vi "main04.vi"() -> ()   [LabVIEW 2018]
uses:
  <vilib>/httpClient/LabVIEWHTTPClient.lvlib
panel:
  in  "탭 컨트롤":enum32{"관심 1", "관심 2", "관심 3", "관심 4", "관심 5"}(tab)
  in  "?":bool
  in  "품   번":string="034220"
  out "거래량":waveform(dbl)(graph)
  out "가격":waveform(i32)(graph)
  out "run":i32
  out "출력":T1
  in  "정지":bool
  in  "정지 2":bool
  out "출력 2":T1
  out "run 2":i32
  out "가격 2":waveform(i32)(graph)
  out "거래량 2":waveform(dbl)(graph)
  in  "품   번 2":string="005290"
  in  "?":bool
  in  "?":bool
  in  "?":bool
  in  "품   번 3":string="042700"
  out "거래량 3":waveform(dbl)(graph)
  out "가격 3":waveform(i32)(graph)
  out "run 3":i32
  out "출력 3":T1
  in  "정지 3":bool
  in  "품   번 4":string="046890"
  out "거래량 4":waveform(dbl)(graph)
  out "가격 4":waveform(i32)(graph)
  out "run 4":i32
  out "출력 4":T1
  in  "정지 4":bool
  in  "?":bool
  in  "?":bool
  in  "품   번 5":string="357780"
  out "거래량 5":waveform(dbl)(graph)
  out "가격 5":waveform(i32)(graph)
  out "run 5":i32
  out "출력 5":T1
  in  "정지 5":bool
  in  "품   번 6":string="012610"
  out "거래량 6":waveform(dbl)(graph)
  out "가격 6":waveform(i32)(graph)
  out "run 6":i32
  out "출력 6":T1
  in  "정지 6":bool
  in  "품   번 7":string="272450"
  out "거래량 7":waveform(dbl)(graph)
  out "가격 7":waveform(i32)(graph)
  out "run 7":i32
  out "출력 7":T1
  in  "정지 7":bool
  in  "품   번 8":string="003490"
  out "거래량 8":waveform(dbl)(graph)
  out "가격 8":waveform(i32)(graph)
  out "run 8":i32
  out "출력 8":T1
  in  "정지 8":bool
  in  "품   번 9":string="091580"
  out "거래량 9":waveform(dbl)(graph)
  out "가격 9":waveform(i32)(graph)
  out "run 9":i32
  out "출력 9":T1
  in  "정지 9":bool
  in  "품   번 10":string="089980"
  out "거래량 10":waveform(dbl)(graph)
  out "가격 10":waveform(i32)(graph)
  out "run 10":i32
  out "출력 10":T1
  in  "정지 10":bool
  in  "품   번 11":string="005070"
  out "거래량 11":waveform(dbl)(graph)
  out "가격 11":waveform(i32)(graph)
  out "run 11":i32
  out "출력 11":T1
  in  "정지 11":bool
  in  "품   번 12":string="078600"
  out "거래량 12":waveform(dbl)(graph)
  out "가격 12":waveform(i32)(graph)
  out "run 12":i32
  out "출력 12":T1
  in  "정지 12":bool
  in  "?":bool
  in  "?":bool
  in  "?":bool
  in  "?":bool
  in  "?":bool
  in  "?":bool
  in  "품   번 13":string="034220"
  out "거래량 13":waveform(dbl)(graph)
  out "가격 13":waveform(i32)(graph)
  out "run 13":i32
  out "출력 13":T1
  in  "정지 13":bool
  in  "품   번 14":string="039130"
  out "거래량 14":waveform(dbl)(graph)
  out "가격 14":waveform(i32)(graph)
  out "run 14":i32
  out "출력 14":T1
  in  "정지 14":bool
  in  "품   번 15":string="080160"
  out "거래량 15":waveform(dbl)(graph)
  out "가격 15":waveform(i32)(graph)
  out "run 15":i32
  out "출력 15":T1
  in  "정지 15":bool
  in  "품   번 16":string="020560"
  out "거래량 16":waveform(dbl)(graph)
  out "가격 16":waveform(i32)(graph)
  out "run 16":i32
  out "출력 16":T1
  in  "정지 16":bool
  in  "품   번 17":string="272450"
  out "거래량 17":waveform(dbl)(graph)
  out "가격 17":waveform(i32)(graph)
  out "run 17":i32
  out "출력 17":T1
  in  "정지 17":bool
  in  "품   번 18":string="003490"
  out "거래량 18":waveform(dbl)(graph)
  out "가격 18":waveform(i32)(graph)
  out "run 18":i32
  out "출력 18":T1
  in  "정지 18":bool
  in  "?":bool
  in  "?":bool
  in  "?":bool
  in  "?":bool
  in  "?":bool
  in  "?":bool
  in  "품   번 19":string="034220"
  out "거래량 19":waveform(dbl)(graph)
  out "가격 19":waveform(i32)(graph)
  out "run 19":i32
  out "출력 19":T1
  in  "정지 19":bool
  in  "품   번 20":string="034220"
  out "거래량 20":waveform(dbl)(graph)
  out "가격 20":waveform(i32)(graph)
  out "run 20":i32
  out "출력 20":T1
  in  "정지 20":bool
  in  "품   번 21":string="034220"
  out "거래량 21":waveform(dbl)(graph)
  out "가격 21":waveform(i32)(graph)
  out "run 21":i32
  out "출력 21":T1
  in  "정지 21":bool
  in  "품   번 22":string="034220"
  out "거래량 22":waveform(dbl)(graph)
  out "가격 22":waveform(i32)(graph)
  out "run 22":i32
  out "출력 22":T1
  in  "정지 22":bool
  in  "품   번 23":string="034220"
  out "거래량 23":waveform(dbl)(graph)
  out "가격 23":waveform(i32)(graph)
  out "run 23":i32
  out "출력 23":T1
  in  "정지 23":bool
  in  "품   번 24":string="034220"
  out "거래량 24":waveform(dbl)(graph)
  out "가격 24":waveform(i32)(graph)
  out "run 24":i32
  out "출력 24":T1
  in  "정지 24":bool
  in  "?":bool
  in  "?":bool
  in  "?":bool
  in  "?":bool
  in  "?":bool
  in  "?":bool
  in  "품   번 25":string="034220"
  out "거래량 25":waveform(dbl)(graph)
  out "가격 25":waveform(i32)(graph)
  out "run 25":i32
  out "출력 25":T1
  in  "정지 25":bool
  in  "품   번 26":string="034220"
  out "거래량 26":waveform(dbl)(graph)
  out "가격 26":waveform(i32)(graph)
  out "run 26":i32
  out "출력 26":T1
  in  "정지 26":bool
  in  "품   번 27":string="034220"
  out "거래량 27":waveform(dbl)(graph)
  out "가격 27":waveform(i32)(graph)
  out "run 27":i32
  out "출력 27":T1
  in  "정지 27":bool
  in  "품   번 28":string="034220"
  out "거래량 28":waveform(dbl)(graph)
  out "가격 28":waveform(i32)(graph)
  out "run 28":i32
  out "출력 28":T1
  in  "정지 28":bool
  in  "품   번 29":string="034220"
  out "거래량 29":waveform(dbl)(graph)
  out "가격 29":waveform(i32)(graph)
  out "run 29":i32
  out "출력 29":T1
  in  "정지 29":bool
  in  "품   번 30":string="034220"
  out "거래량 30":waveform(dbl)(graph)
  out "가격 30":waveform(i32)(graph)
  out "run 30":i32
  out "출력 30":T1
  in  "정지 30":bool
  in  "?":bool
  in  "?":bool
  in  "?":bool
  in  "?":bool
  in  "?":bool
  in  "?":bool
  # "Naver 주식 데이터 가져오기"
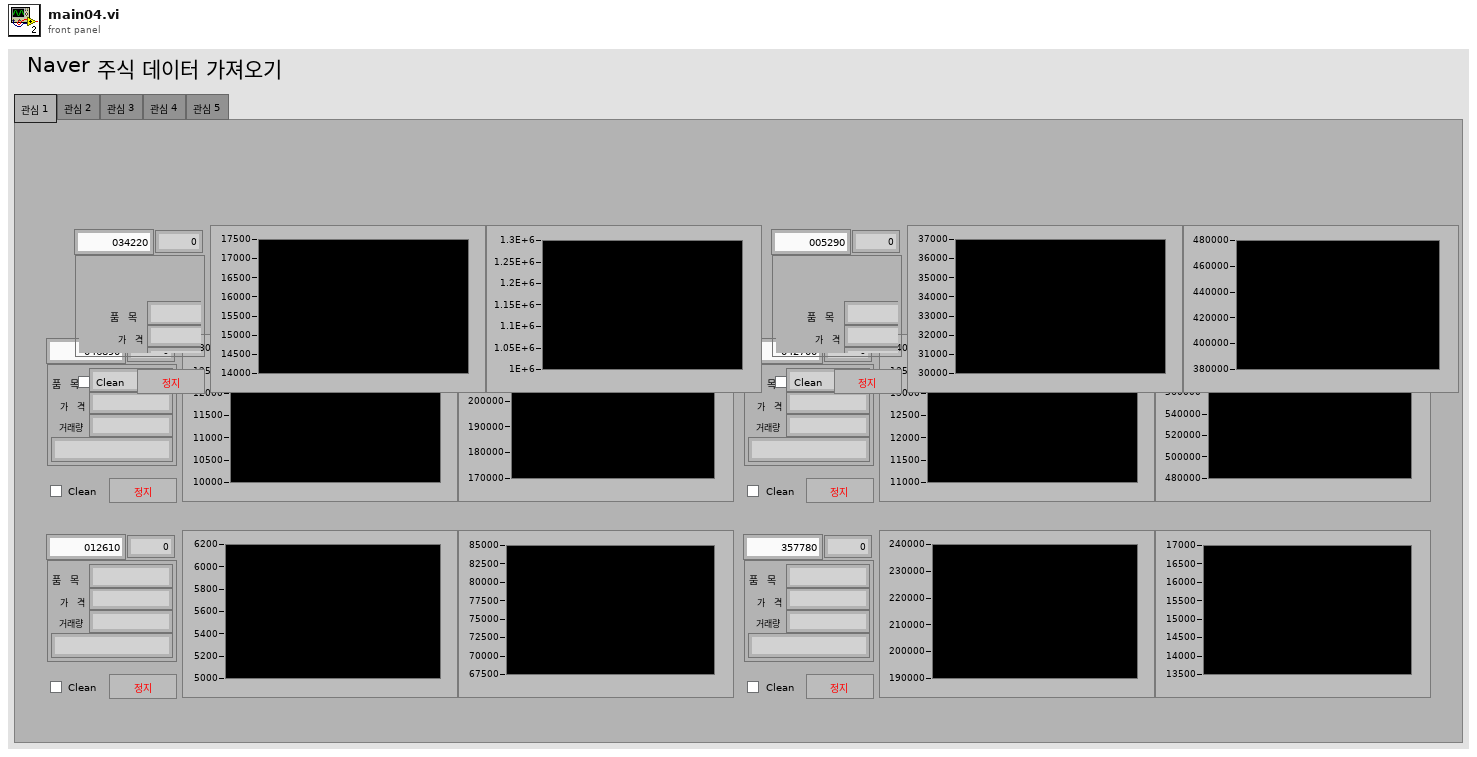
[diagram p1: front panel]
types:
  T1 = cluster{"품   목":string, "가   격":i32, "거래량":dbl, "일시":string}
  T2 = typedef "LabVIEWHTTPClient.lvlib/ClientHandle.ctl" = refnum<k1>
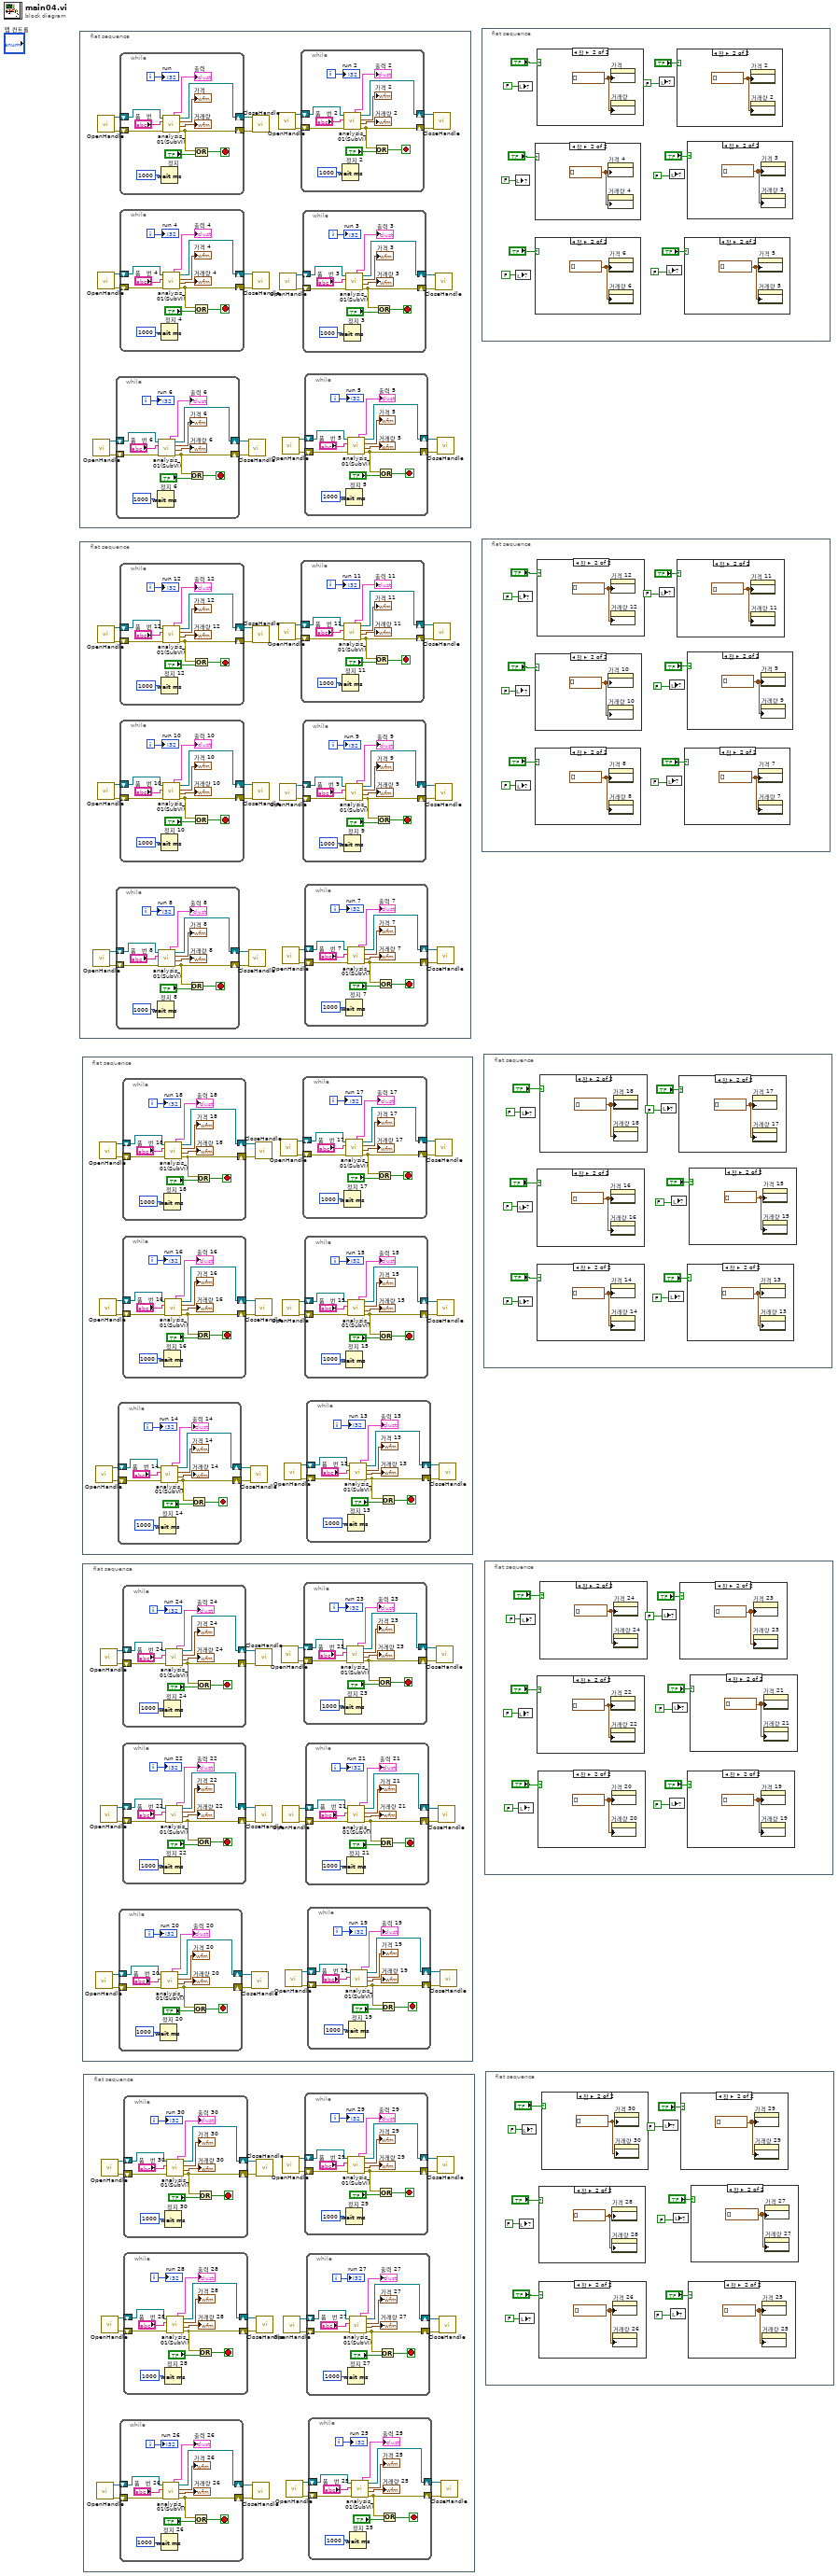
[diagram p0: block diagram]
diagram:
  n1 = flat-sequence {
    frame #0 {
      n2 = call <vilib>:"OpenHandle.vi"() -> ("client handle out"=w5:T2, "error out"=w6:errorcluster)  [unwired: 14 in]
      n3 = call <vilib>:"OpenHandle.vi"() -> ("client handle out"=w21:T2, "error out"=w22:errorcluster)  [unwired: 14 in]
      n4 = call <vilib>:"OpenHandle.vi"() -> ("client handle out"=w12:T2, "error out"=w11:errorcluster)  [unwired: 14 in]
      n5 = while {
        shift-right: [w46] -> w7
        shift-left: w5 -> [w47]
        shift-right: [w44] -> w8
        shift-left: w6 -> [w45]
        i -> [w41]
        stop <- w42 stop-if-true
        n6 = Wait (ms)(milliseconds to wait=u32 1000 ("대기 시간 (ms)")) -> ()  [unwired: 1 out]
        n7 = call "analysis_01(SubVI).vi"("에러 입력(에러 없음)"=w45, "품   번"="품   번 6", "참조 번호 입력"=w47) -> ("에러 출력"=w44:errorcluster, "거래량"=→"거래량 6":waveform(dbl), "가격"=→"가격 6":waveform(i32), "참조 번호 출력"=w46:T2, "출력"=→"출력 6":T1)  [unwired: 4 in]
        n8 = Or(x=w44, y="정지 6") -> (x .or. y?=w42:bool)
        "run 6" <- w41
      }
      n9 = while {
        shift-right: [w94] -> w23
        shift-left: w21 -> [w95]
        shift-right: [w92] -> w24
        shift-left: w22 -> [w93]
        i -> [w89]
        stop <- w90 stop-if-true
        n10 = Wait (ms)(milliseconds to wait=u32 1000 ("대기 시간 (ms)")) -> ()  [unwired: 1 out]
        n11 = call "analysis_01(SubVI).vi"("에러 입력(에러 없음)"=w93, "품   번"="품   번", "참조 번호 입력"=w95) -> ("에러 출력"=w92:errorcluster, "거래량"=→"거래량":waveform(dbl), "가격"=→"가격":waveform(i32), "참조 번호 출력"=w94:T2, "출력"=→"출력":T1)  [unwired: 4 in]
        n12 = Or(x=w92, y="정지") -> (x .or. y?=w90:bool)
        "run" <- w89
      }
      n13 = while {
        shift-right: [w70] -> w10
        shift-left: w12 -> [w71]
        shift-right: [w68] -> w9
        shift-left: w11 -> [w69]
        i -> [w65]
        stop <- w66 stop-if-true
        n14 = Wait (ms)(milliseconds to wait=u32 1000 ("대기 시간 (ms)")) -> ()  [unwired: 1 out]
        n15 = call "analysis_01(SubVI).vi"("에러 입력(에러 없음)"=w69, "품   번"="품   번 4", "참조 번호 입력"=w71) -> ("에러 출력"=w68:errorcluster, "거래량"=→"거래량 4":waveform(dbl), "가격"=→"가격 4":waveform(i32), "참조 번호 출력"=w70:T2, "출력"=→"출력 4":T1)  [unwired: 4 in]
        n16 = Or(x=w68, y="정지 4") -> (x .or. y?=w66:bool)
        "run 4" <- w65
      }
      n17 = call <vilib>:"CloseHandle.vi"("client handle"=w7, "error in (no error)"=w8) -> ()  [unwired: 13 in, 1 out]
      n18 = call <vilib>:"CloseHandle.vi"("client handle"=w23, "error in (no error)"=w24) -> ()  [unwired: 13 in, 1 out]
      n19 = call <vilib>:"CloseHandle.vi"("client handle"=w10, "error in (no error)"=w9) -> ()  [unwired: 13 in, 1 out]
      n20 = call <vilib>:"OpenHandle.vi"() -> ("client handle out"=w20:T2, "error out"=w19:errorcluster)  [unwired: 14 in]
      n21 = call <vilib>:"OpenHandle.vi"() -> ("client handle out"=w13:T2, "error out"=w14:errorcluster)  [unwired: 14 in]
      n22 = call <vilib>:"OpenHandle.vi"() -> ("client handle out"=w4:T2, "error out"=w3:errorcluster)  [unwired: 14 in]
      n23 = while {
        shift-right: [w82] -> w18
        shift-left: w20 -> [w83]
        shift-right: [w80] -> w17
        shift-left: w19 -> [w81]
        i -> [w77]
        stop <- w78 stop-if-true
        n24 = Wait (ms)(milliseconds to wait=u32 1000 ("대기 시간 (ms)")) -> ()  [unwired: 1 out]
        n25 = call "analysis_01(SubVI).vi"("에러 입력(에러 없음)"=w81, "품   번"="품   번 2", "참조 번호 입력"=w83) -> ("에러 출력"=w80:errorcluster, "거래량"=→"거래량 2":waveform(dbl), "가격"=→"가격 2":waveform(i32), "참조 번호 출력"=w82:T2, "출력"=→"출력 2":T1)  [unwired: 4 in]
        n26 = Or(x=w80, y="정지 2") -> (x .or. y?=w78:bool)
        "run 2" <- w77
      }
      n27 = while {
        shift-right: [w58] -> w15
        shift-left: w13 -> [w59]
        shift-right: [w56] -> w16
        shift-left: w14 -> [w57]
        i -> [w53]
        stop <- w54 stop-if-true
        n28 = Wait (ms)(milliseconds to wait=u32 1000 ("대기 시간 (ms)")) -> ()  [unwired: 1 out]
        n29 = call "analysis_01(SubVI).vi"("에러 입력(에러 없음)"=w57, "품   번"="품   번 3", "참조 번호 입력"=w59) -> ("에러 출력"=w56:errorcluster, "거래량"=→"거래량 3":waveform(dbl), "가격"=→"가격 3":waveform(i32), "참조 번호 출력"=w58:T2, "출력"=→"출력 3":T1)  [unwired: 4 in]
        n30 = Or(x=w56, y="정지 3") -> (x .or. y?=w54:bool)
        "run 3" <- w53
      }
      n31 = while {
        shift-right: [w34] -> w2
        shift-left: w4 -> [w35]
        shift-right: [w32] -> w1
        shift-left: w3 -> [w33]
        i -> [w29]
        stop <- w30 stop-if-true
        n32 = Wait (ms)(milliseconds to wait=u32 1000 ("대기 시간 (ms)")) -> ()  [unwired: 1 out]
        n33 = call "analysis_01(SubVI).vi"("에러 입력(에러 없음)"=w33, "품   번"="품   번 5", "참조 번호 입력"=w35) -> ("에러 출력"=w32:errorcluster, "거래량"=→"거래량 5":waveform(dbl), "가격"=→"가격 5":waveform(i32), "참조 번호 출력"=w34:T2, "출력"=→"출력 5":T1)  [unwired: 4 in]
        n34 = Or(x=w32, y="정지 5") -> (x .or. y?=w30:bool)
        "run 5" <- w29
      }
      n35 = call <vilib>:"CloseHandle.vi"("client handle"=w18, "error in (no error)"=w17) -> ()  [unwired: 13 in, 1 out]
      n36 = call <vilib>:"CloseHandle.vi"("client handle"=w15, "error in (no error)"=w16) -> ()  [unwired: 13 in, 1 out]
      n37 = call <vilib>:"CloseHandle.vi"("client handle"=w2, "error in (no error)"=w1) -> ()  [unwired: 13 in, 1 out]
    }
  }
  n38 = flat-sequence {
    frame #0 {
      n39 = call <vilib>:"OpenHandle.vi"() -> ("client handle out"=w101:T2, "error out"=w102:errorcluster)  [unwired: 14 in]
      n40 = call <vilib>:"OpenHandle.vi"() -> ("client handle out"=w117:T2, "error out"=w118:errorcluster)  [unwired: 14 in]
      n41 = call <vilib>:"OpenHandle.vi"() -> ("client handle out"=w108:T2, "error out"=w107:errorcluster)  [unwired: 14 in]
      n42 = while {
        shift-right: [w142] -> w103
        shift-left: w101 -> [w143]
        shift-right: [w140] -> w104
        shift-left: w102 -> [w141]
        i -> [w137]
        stop <- w138 stop-if-true
        n43 = Wait (ms)(milliseconds to wait=u32 1000 ("대기 시간 (ms)")) -> ()  [unwired: 1 out]
        n44 = call "analysis_01(SubVI).vi"("에러 입력(에러 없음)"=w141, "품   번"="품   번 8", "참조 번호 입력"=w143) -> ("에러 출력"=w140:errorcluster, "거래량"=→"거래량 8":waveform(dbl), "가격"=→"가격 8":waveform(i32), "참조 번호 출력"=w142:T2, "출력"=→"출력 8":T1)  [unwired: 4 in]
        n45 = Or(x=w140, y="정지 8") -> (x .or. y?=w138:bool)
        "run 8" <- w137
      }
      n46 = while {
        shift-right: [w190] -> w119
        shift-left: w117 -> [w191]
        shift-right: [w188] -> w120
        shift-left: w118 -> [w189]
        i -> [w185]
        stop <- w186 stop-if-true
        n47 = Wait (ms)(milliseconds to wait=u32 1000 ("대기 시간 (ms)")) -> ()  [unwired: 1 out]
        n48 = call "analysis_01(SubVI).vi"("에러 입력(에러 없음)"=w189, "품   번"="품   번 12", "참조 번호 입력"=w191) -> ("에러 출력"=w188:errorcluster, "거래량"=→"거래량 12":waveform(dbl), "가격"=→"가격 12":waveform(i32), "참조 번호 출력"=w190:T2, "출력"=→"출력 12":T1)  [unwired: 4 in]
        n49 = Or(x=w188, y="정지 12") -> (x .or. y?=w186:bool)
        "run 12" <- w185
      }
      n50 = while {
        shift-right: [w166] -> w106
        shift-left: w108 -> [w167]
        shift-right: [w164] -> w105
        shift-left: w107 -> [w165]
        i -> [w161]
        stop <- w162 stop-if-true
        n51 = Wait (ms)(milliseconds to wait=u32 1000 ("대기 시간 (ms)")) -> ()  [unwired: 1 out]
        n52 = call "analysis_01(SubVI).vi"("에러 입력(에러 없음)"=w165, "품   번"="품   번 10", "참조 번호 입력"=w167) -> ("에러 출력"=w164:errorcluster, "거래량"=→"거래량 10":waveform(dbl), "가격"=→"가격 10":waveform(i32), "참조 번호 출력"=w166:T2, "출력"=→"출력 10":T1)  [unwired: 4 in]
        n53 = Or(x=w164, y="정지 10") -> (x .or. y?=w162:bool)
        "run 10" <- w161
      }
      n54 = call <vilib>:"CloseHandle.vi"("client handle"=w103, "error in (no error)"=w104) -> ()  [unwired: 13 in, 1 out]
      n55 = call <vilib>:"CloseHandle.vi"("client handle"=w119, "error in (no error)"=w120) -> ()  [unwired: 13 in, 1 out]
      n56 = call <vilib>:"CloseHandle.vi"("client handle"=w106, "error in (no error)"=w105) -> ()  [unwired: 13 in, 1 out]
      n57 = call <vilib>:"OpenHandle.vi"() -> ("client handle out"=w116:T2, "error out"=w115:errorcluster)  [unwired: 14 in]
      n58 = call <vilib>:"OpenHandle.vi"() -> ("client handle out"=w109:T2, "error out"=w110:errorcluster)  [unwired: 14 in]
      n59 = call <vilib>:"OpenHandle.vi"() -> ("client handle out"=w100:T2, "error out"=w99:errorcluster)  [unwired: 14 in]
      n60 = while {
        shift-right: [w178] -> w114
        shift-left: w116 -> [w179]
        shift-right: [w176] -> w113
        shift-left: w115 -> [w177]
        i -> [w173]
        stop <- w174 stop-if-true
        n61 = Wait (ms)(milliseconds to wait=u32 1000 ("대기 시간 (ms)")) -> ()  [unwired: 1 out]
        n62 = call "analysis_01(SubVI).vi"("에러 입력(에러 없음)"=w177, "품   번"="품   번 11", "참조 번호 입력"=w179) -> ("에러 출력"=w176:errorcluster, "거래량"=→"거래량 11":waveform(dbl), "가격"=→"가격 11":waveform(i32), "참조 번호 출력"=w178:T2, "출력"=→"출력 11":T1)  [unwired: 4 in]
        n63 = Or(x=w176, y="정지 11") -> (x .or. y?=w174:bool)
        "run 11" <- w173
      }
      n64 = while {
        shift-right: [w154] -> w111
        shift-left: w109 -> [w155]
        shift-right: [w152] -> w112
        shift-left: w110 -> [w153]
        i -> [w149]
        stop <- w150 stop-if-true
        n65 = Wait (ms)(milliseconds to wait=u32 1000 ("대기 시간 (ms)")) -> ()  [unwired: 1 out]
        n66 = call "analysis_01(SubVI).vi"("에러 입력(에러 없음)"=w153, "품   번"="품   번 9", "참조 번호 입력"=w155) -> ("에러 출력"=w152:errorcluster, "거래량"=→"거래량 9":waveform(dbl), "가격"=→"가격 9":waveform(i32), "참조 번호 출력"=w154:T2, "출력"=→"출력 9":T1)  [unwired: 4 in]
        n67 = Or(x=w152, y="정지 9") -> (x .or. y?=w150:bool)
        "run 9" <- w149
      }
      n68 = while {
        shift-right: [w130] -> w98
        shift-left: w100 -> [w131]
        shift-right: [w128] -> w97
        shift-left: w99 -> [w129]
        i -> [w125]
        stop <- w126 stop-if-true
        n69 = Wait (ms)(milliseconds to wait=u32 1000 ("대기 시간 (ms)")) -> ()  [unwired: 1 out]
        n70 = call "analysis_01(SubVI).vi"("에러 입력(에러 없음)"=w129, "품   번"="품   번 7", "참조 번호 입력"=w131) -> ("에러 출력"=w128:errorcluster, "거래량"=→"거래량 7":waveform(dbl), "가격"=→"가격 7":waveform(i32), "참조 번호 출력"=w130:T2, "출력"=→"출력 7":T1)  [unwired: 4 in]
        n71 = Or(x=w128, y="정지 7") -> (x .or. y?=w126:bool)
        "run 7" <- w125
      }
      n72 = call <vilib>:"CloseHandle.vi"("client handle"=w114, "error in (no error)"=w113) -> ()  [unwired: 13 in, 1 out]
      n73 = call <vilib>:"CloseHandle.vi"("client handle"=w111, "error in (no error)"=w112) -> ()  [unwired: 13 in, 1 out]
      n74 = call <vilib>:"CloseHandle.vi"("client handle"=w98, "error in (no error)"=w97) -> ()  [unwired: 13 in, 1 out]
    }
  }
  n75 = flat-sequence {
    frame #0 {
      n76 = call <vilib>:"OpenHandle.vi"() -> ("client handle out"=w197:T2, "error out"=w198:errorcluster)  [unwired: 14 in]
      n77 = call <vilib>:"OpenHandle.vi"() -> ("client handle out"=w213:T2, "error out"=w214:errorcluster)  [unwired: 14 in]
      n78 = call <vilib>:"OpenHandle.vi"() -> ("client handle out"=w204:T2, "error out"=w203:errorcluster)  [unwired: 14 in]
      n79 = while {
        shift-right: [w238] -> w199
        shift-left: w197 -> [w239]
        shift-right: [w236] -> w200
        shift-left: w198 -> [w237]
        i -> [w233]
        stop <- w234 stop-if-true
        n80 = Wait (ms)(milliseconds to wait=u32 1000 ("대기 시간 (ms)")) -> ()  [unwired: 1 out]
        n81 = call "analysis_01(SubVI).vi"("에러 입력(에러 없음)"=w237, "품   번"="품   번 14", "참조 번호 입력"=w239) -> ("에러 출력"=w236:errorcluster, "거래량"=→"거래량 14":waveform(dbl), "가격"=→"가격 14":waveform(i32), "참조 번호 출력"=w238:T2, "출력"=→"출력 14":T1)  [unwired: 4 in]
        n82 = Or(x=w236, y="정지 14") -> (x .or. y?=w234:bool)
        "run 14" <- w233
      }
      n83 = while {
        shift-right: [w286] -> w215
        shift-left: w213 -> [w287]
        shift-right: [w284] -> w216
        shift-left: w214 -> [w285]
        i -> [w281]
        stop <- w282 stop-if-true
        n84 = Wait (ms)(milliseconds to wait=u32 1000 ("대기 시간 (ms)")) -> ()  [unwired: 1 out]
        n85 = call "analysis_01(SubVI).vi"("에러 입력(에러 없음)"=w285, "품   번"="품   번 18", "참조 번호 입력"=w287) -> ("에러 출력"=w284:errorcluster, "거래량"=→"거래량 18":waveform(dbl), "가격"=→"가격 18":waveform(i32), "참조 번호 출력"=w286:T2, "출력"=→"출력 18":T1)  [unwired: 4 in]
        n86 = Or(x=w284, y="정지 18") -> (x .or. y?=w282:bool)
        "run 18" <- w281
      }
      n87 = while {
        shift-right: [w262] -> w202
        shift-left: w204 -> [w263]
        shift-right: [w260] -> w201
        shift-left: w203 -> [w261]
        i -> [w257]
        stop <- w258 stop-if-true
        n88 = Wait (ms)(milliseconds to wait=u32 1000 ("대기 시간 (ms)")) -> ()  [unwired: 1 out]
        n89 = call "analysis_01(SubVI).vi"("에러 입력(에러 없음)"=w261, "품   번"="품   번 16", "참조 번호 입력"=w263) -> ("에러 출력"=w260:errorcluster, "거래량"=→"거래량 16":waveform(dbl), "가격"=→"가격 16":waveform(i32), "참조 번호 출력"=w262:T2, "출력"=→"출력 16":T1)  [unwired: 4 in]
        n90 = Or(x=w260, y="정지 16") -> (x .or. y?=w258:bool)
        "run 16" <- w257
      }
      n91 = call <vilib>:"CloseHandle.vi"("client handle"=w199, "error in (no error)"=w200) -> ()  [unwired: 13 in, 1 out]
      n92 = call <vilib>:"CloseHandle.vi"("client handle"=w215, "error in (no error)"=w216) -> ()  [unwired: 13 in, 1 out]
      n93 = call <vilib>:"CloseHandle.vi"("client handle"=w202, "error in (no error)"=w201) -> ()  [unwired: 13 in, 1 out]
      n94 = call <vilib>:"OpenHandle.vi"() -> ("client handle out"=w212:T2, "error out"=w211:errorcluster)  [unwired: 14 in]
      n95 = call <vilib>:"OpenHandle.vi"() -> ("client handle out"=w205:T2, "error out"=w206:errorcluster)  [unwired: 14 in]
      n96 = call <vilib>:"OpenHandle.vi"() -> ("client handle out"=w196:T2, "error out"=w195:errorcluster)  [unwired: 14 in]
      n97 = while {
        shift-right: [w274] -> w210
        shift-left: w212 -> [w275]
        shift-right: [w272] -> w209
        shift-left: w211 -> [w273]
        i -> [w269]
        stop <- w270 stop-if-true
        n98 = Wait (ms)(milliseconds to wait=u32 1000 ("대기 시간 (ms)")) -> ()  [unwired: 1 out]
        n99 = call "analysis_01(SubVI).vi"("에러 입력(에러 없음)"=w273, "품   번"="품   번 17", "참조 번호 입력"=w275) -> ("에러 출력"=w272:errorcluster, "거래량"=→"거래량 17":waveform(dbl), "가격"=→"가격 17":waveform(i32), "참조 번호 출력"=w274:T2, "출력"=→"출력 17":T1)  [unwired: 4 in]
        n100 = Or(x=w272, y="정지 17") -> (x .or. y?=w270:bool)
        "run 17" <- w269
      }
      n101 = while {
        shift-right: [w250] -> w207
        shift-left: w205 -> [w251]
        shift-right: [w248] -> w208
        shift-left: w206 -> [w249]
        i -> [w245]
        stop <- w246 stop-if-true
        n102 = Wait (ms)(milliseconds to wait=u32 1000 ("대기 시간 (ms)")) -> ()  [unwired: 1 out]
        n103 = call "analysis_01(SubVI).vi"("에러 입력(에러 없음)"=w249, "품   번"="품   번 15", "참조 번호 입력"=w251) -> ("에러 출력"=w248:errorcluster, "거래량"=→"거래량 15":waveform(dbl), "가격"=→"가격 15":waveform(i32), "참조 번호 출력"=w250:T2, "출력"=→"출력 15":T1)  [unwired: 4 in]
        n104 = Or(x=w248, y="정지 15") -> (x .or. y?=w246:bool)
        "run 15" <- w245
      }
      n105 = while {
        shift-right: [w226] -> w194
        shift-left: w196 -> [w227]
        shift-right: [w224] -> w193
        shift-left: w195 -> [w225]
        i -> [w221]
        stop <- w222 stop-if-true
        n106 = Wait (ms)(milliseconds to wait=u32 1000 ("대기 시간 (ms)")) -> ()  [unwired: 1 out]
        n107 = call "analysis_01(SubVI).vi"("에러 입력(에러 없음)"=w225, "품   번"="품   번 13", "참조 번호 입력"=w227) -> ("에러 출력"=w224:errorcluster, "거래량"=→"거래량 13":waveform(dbl), "가격"=→"가격 13":waveform(i32), "참조 번호 출력"=w226:T2, "출력"=→"출력 13":T1)  [unwired: 4 in]
        n108 = Or(x=w224, y="정지 13") -> (x .or. y?=w222:bool)
        "run 13" <- w221
      }
      n109 = call <vilib>:"CloseHandle.vi"("client handle"=w210, "error in (no error)"=w209) -> ()  [unwired: 13 in, 1 out]
      n110 = call <vilib>:"CloseHandle.vi"("client handle"=w207, "error in (no error)"=w208) -> ()  [unwired: 13 in, 1 out]
      n111 = call <vilib>:"CloseHandle.vi"("client handle"=w194, "error in (no error)"=w193) -> ()  [unwired: 13 in, 1 out]
    }
  }
  n112 = flat-sequence {
    frame #0 {
      n113 = call <vilib>:"OpenHandle.vi"() -> ("client handle out"=w293:T2, "error out"=w294:errorcluster)  [unwired: 14 in]
      n114 = call <vilib>:"OpenHandle.vi"() -> ("client handle out"=w309:T2, "error out"=w310:errorcluster)  [unwired: 14 in]
      n115 = call <vilib>:"OpenHandle.vi"() -> ("client handle out"=w300:T2, "error out"=w299:errorcluster)  [unwired: 14 in]
      n116 = while {
        shift-right: [w334] -> w295
        shift-left: w293 -> [w335]
        shift-right: [w332] -> w296
        shift-left: w294 -> [w333]
        i -> [w329]
        stop <- w330 stop-if-true
        n117 = Wait (ms)(milliseconds to wait=u32 1000 ("대기 시간 (ms)")) -> ()  [unwired: 1 out]
        n118 = call "analysis_01(SubVI).vi"("에러 입력(에러 없음)"=w333, "품   번"="품   번 20", "참조 번호 입력"=w335) -> ("에러 출력"=w332:errorcluster, "거래량"=→"거래량 20":waveform(dbl), "가격"=→"가격 20":waveform(i32), "참조 번호 출력"=w334:T2, "출력"=→"출력 20":T1)  [unwired: 4 in]
        n119 = Or(x=w332, y="정지 20") -> (x .or. y?=w330:bool)
        "run 20" <- w329
      }
      n120 = while {
        shift-right: [w382] -> w311
        shift-left: w309 -> [w383]
        shift-right: [w380] -> w312
        shift-left: w310 -> [w381]
        i -> [w377]
        stop <- w378 stop-if-true
        n121 = Wait (ms)(milliseconds to wait=u32 1000 ("대기 시간 (ms)")) -> ()  [unwired: 1 out]
        n122 = call "analysis_01(SubVI).vi"("에러 입력(에러 없음)"=w381, "품   번"="품   번 24", "참조 번호 입력"=w383) -> ("에러 출력"=w380:errorcluster, "거래량"=→"거래량 24":waveform(dbl), "가격"=→"가격 24":waveform(i32), "참조 번호 출력"=w382:T2, "출력"=→"출력 24":T1)  [unwired: 4 in]
        n123 = Or(x=w380, y="정지 24") -> (x .or. y?=w378:bool)
        "run 24" <- w377
      }
      n124 = while {
        shift-right: [w358] -> w298
        shift-left: w300 -> [w359]
        shift-right: [w356] -> w297
        shift-left: w299 -> [w357]
        i -> [w353]
        stop <- w354 stop-if-true
        n125 = Wait (ms)(milliseconds to wait=u32 1000 ("대기 시간 (ms)")) -> ()  [unwired: 1 out]
        n126 = call "analysis_01(SubVI).vi"("에러 입력(에러 없음)"=w357, "품   번"="품   번 22", "참조 번호 입력"=w359) -> ("에러 출력"=w356:errorcluster, "거래량"=→"거래량 22":waveform(dbl), "가격"=→"가격 22":waveform(i32), "참조 번호 출력"=w358:T2, "출력"=→"출력 22":T1)  [unwired: 4 in]
        n127 = Or(x=w356, y="정지 22") -> (x .or. y?=w354:bool)
        "run 22" <- w353
      }
      n128 = call <vilib>:"CloseHandle.vi"("client handle"=w295, "error in (no error)"=w296) -> ()  [unwired: 13 in, 1 out]
      n129 = call <vilib>:"CloseHandle.vi"("client handle"=w311, "error in (no error)"=w312) -> ()  [unwired: 13 in, 1 out]
      n130 = call <vilib>:"CloseHandle.vi"("client handle"=w298, "error in (no error)"=w297) -> ()  [unwired: 13 in, 1 out]
      n131 = call <vilib>:"OpenHandle.vi"() -> ("client handle out"=w308:T2, "error out"=w307:errorcluster)  [unwired: 14 in]
      n132 = call <vilib>:"OpenHandle.vi"() -> ("client handle out"=w301:T2, "error out"=w302:errorcluster)  [unwired: 14 in]
      n133 = call <vilib>:"OpenHandle.vi"() -> ("client handle out"=w292:T2, "error out"=w291:errorcluster)  [unwired: 14 in]
      n134 = while {
        shift-right: [w370] -> w306
        shift-left: w308 -> [w371]
        shift-right: [w368] -> w305
        shift-left: w307 -> [w369]
        i -> [w365]
        stop <- w366 stop-if-true
        n135 = Wait (ms)(milliseconds to wait=u32 1000 ("대기 시간 (ms)")) -> ()  [unwired: 1 out]
        n136 = call "analysis_01(SubVI).vi"("에러 입력(에러 없음)"=w369, "품   번"="품   번 23", "참조 번호 입력"=w371) -> ("에러 출력"=w368:errorcluster, "거래량"=→"거래량 23":waveform(dbl), "가격"=→"가격 23":waveform(i32), "참조 번호 출력"=w370:T2, "출력"=→"출력 23":T1)  [unwired: 4 in]
        n137 = Or(x=w368, y="정지 23") -> (x .or. y?=w366:bool)
        "run 23" <- w365
      }
      n138 = while {
        shift-right: [w346] -> w303
        shift-left: w301 -> [w347]
        shift-right: [w344] -> w304
        shift-left: w302 -> [w345]
        i -> [w341]
        stop <- w342 stop-if-true
        n139 = Wait (ms)(milliseconds to wait=u32 1000 ("대기 시간 (ms)")) -> ()  [unwired: 1 out]
        n140 = call "analysis_01(SubVI).vi"("에러 입력(에러 없음)"=w345, "품   번"="품   번 21", "참조 번호 입력"=w347) -> ("에러 출력"=w344:errorcluster, "거래량"=→"거래량 21":waveform(dbl), "가격"=→"가격 21":waveform(i32), "참조 번호 출력"=w346:T2, "출력"=→"출력 21":T1)  [unwired: 4 in]
        n141 = Or(x=w344, y="정지 21") -> (x .or. y?=w342:bool)
        "run 21" <- w341
      }
      n142 = while {
        shift-right: [w322] -> w290
        shift-left: w292 -> [w323]
        shift-right: [w320] -> w289
        shift-left: w291 -> [w321]
        i -> [w317]
        stop <- w318 stop-if-true
        n143 = Wait (ms)(milliseconds to wait=u32 1000 ("대기 시간 (ms)")) -> ()  [unwired: 1 out]
        n144 = call "analysis_01(SubVI).vi"("에러 입력(에러 없음)"=w321, "품   번"="품   번 19", "참조 번호 입력"=w323) -> ("에러 출력"=w320:errorcluster, "거래량"=→"거래량 19":waveform(dbl), "가격"=→"가격 19":waveform(i32), "참조 번호 출력"=w322:T2, "출력"=→"출력 19":T1)  [unwired: 4 in]
        n145 = Or(x=w320, y="정지 19") -> (x .or. y?=w318:bool)
        "run 19" <- w317
      }
      n146 = call <vilib>:"CloseHandle.vi"("client handle"=w306, "error in (no error)"=w305) -> ()  [unwired: 13 in, 1 out]
      n147 = call <vilib>:"CloseHandle.vi"("client handle"=w303, "error in (no error)"=w304) -> ()  [unwired: 13 in, 1 out]
      n148 = call <vilib>:"CloseHandle.vi"("client handle"=w290, "error in (no error)"=w289) -> ()  [unwired: 13 in, 1 out]
    }
  }
  n149 = flat-sequence {
    frame #0 {
      n150 = call <vilib>:"OpenHandle.vi"() -> ("client handle out"=w389:T2, "error out"=w390:errorcluster)  [unwired: 14 in]
      n151 = call <vilib>:"OpenHandle.vi"() -> ("client handle out"=w405:T2, "error out"=w406:errorcluster)  [unwired: 14 in]
      n152 = call <vilib>:"OpenHandle.vi"() -> ("client handle out"=w396:T2, "error out"=w395:errorcluster)  [unwired: 14 in]
      n153 = while {
        shift-right: [w430] -> w391
        shift-left: w389 -> [w431]
        shift-right: [w428] -> w392
        shift-left: w390 -> [w429]
        i -> [w425]
        stop <- w426 stop-if-true
        n154 = Wait (ms)(milliseconds to wait=u32 1000 ("대기 시간 (ms)")) -> ()  [unwired: 1 out]
        n155 = call "analysis_01(SubVI).vi"("에러 입력(에러 없음)"=w429, "품   번"="품   번 26", "참조 번호 입력"=w431) -> ("에러 출력"=w428:errorcluster, "거래량"=→"거래량 26":waveform(dbl), "가격"=→"가격 26":waveform(i32), "참조 번호 출력"=w430:T2, "출력"=→"출력 26":T1)  [unwired: 4 in]
        n156 = Or(x=w428, y="정지 26") -> (x .or. y?=w426:bool)
        "run 26" <- w425
      }
      n157 = while {
        shift-right: [w478] -> w407
        shift-left: w405 -> [w479]
        shift-right: [w476] -> w408
        shift-left: w406 -> [w477]
        i -> [w473]
        stop <- w474 stop-if-true
        n158 = Wait (ms)(milliseconds to wait=u32 1000 ("대기 시간 (ms)")) -> ()  [unwired: 1 out]
        n159 = call "analysis_01(SubVI).vi"("에러 입력(에러 없음)"=w477, "품   번"="품   번 30", "참조 번호 입력"=w479) -> ("에러 출력"=w476:errorcluster, "거래량"=→"거래량 30":waveform(dbl), "가격"=→"가격 30":waveform(i32), "참조 번호 출력"=w478:T2, "출력"=→"출력 30":T1)  [unwired: 4 in]
        n160 = Or(x=w476, y="정지 30") -> (x .or. y?=w474:bool)
        "run 30" <- w473
      }
      n161 = while {
        shift-right: [w454] -> w394
        shift-left: w396 -> [w455]
        shift-right: [w452] -> w393
        shift-left: w395 -> [w453]
        i -> [w449]
        stop <- w450 stop-if-true
        n162 = Wait (ms)(milliseconds to wait=u32 1000 ("대기 시간 (ms)")) -> ()  [unwired: 1 out]
        n163 = call "analysis_01(SubVI).vi"("에러 입력(에러 없음)"=w453, "품   번"="품   번 28", "참조 번호 입력"=w455) -> ("에러 출력"=w452:errorcluster, "거래량"=→"거래량 28":waveform(dbl), "가격"=→"가격 28":waveform(i32), "참조 번호 출력"=w454:T2, "출력"=→"출력 28":T1)  [unwired: 4 in]
        n164 = Or(x=w452, y="정지 28") -> (x .or. y?=w450:bool)
        "run 28" <- w449
      }
      n165 = call <vilib>:"CloseHandle.vi"("client handle"=w391, "error in (no error)"=w392) -> ()  [unwired: 13 in, 1 out]
      n166 = call <vilib>:"CloseHandle.vi"("client handle"=w407, "error in (no error)"=w408) -> ()  [unwired: 13 in, 1 out]
      n167 = call <vilib>:"CloseHandle.vi"("client handle"=w394, "error in (no error)"=w393) -> ()  [unwired: 13 in, 1 out]
      n168 = call <vilib>:"OpenHandle.vi"() -> ("client handle out"=w404:T2, "error out"=w403:errorcluster)  [unwired: 14 in]
      n169 = call <vilib>:"OpenHandle.vi"() -> ("client handle out"=w397:T2, "error out"=w398:errorcluster)  [unwired: 14 in]
      n170 = call <vilib>:"OpenHandle.vi"() -> ("client handle out"=w388:T2, "error out"=w387:errorcluster)  [unwired: 14 in]
      n171 = while {
        shift-right: [w466] -> w402
        shift-left: w404 -> [w467]
        shift-right: [w464] -> w401
        shift-left: w403 -> [w465]
        i -> [w461]
        stop <- w462 stop-if-true
        n172 = Wait (ms)(milliseconds to wait=u32 1000 ("대기 시간 (ms)")) -> ()  [unwired: 1 out]
        n173 = call "analysis_01(SubVI).vi"("에러 입력(에러 없음)"=w465, "품   번"="품   번 29", "참조 번호 입력"=w467) -> ("에러 출력"=w464:errorcluster, "거래량"=→"거래량 29":waveform(dbl), "가격"=→"가격 29":waveform(i32), "참조 번호 출력"=w466:T2, "출력"=→"출력 29":T1)  [unwired: 4 in]
        n174 = Or(x=w464, y="정지 29") -> (x .or. y?=w462:bool)
        "run 29" <- w461
      }
      n175 = while {
        shift-right: [w442] -> w399
        shift-left: w397 -> [w443]
        shift-right: [w440] -> w400
        shift-left: w398 -> [w441]
        i -> [w437]
        stop <- w438 stop-if-true
        n176 = Wait (ms)(milliseconds to wait=u32 1000 ("대기 시간 (ms)")) -> ()  [unwired: 1 out]
        n177 = call "analysis_01(SubVI).vi"("에러 입력(에러 없음)"=w441, "품   번"="품   번 27", "참조 번호 입력"=w443) -> ("에러 출력"=w440:errorcluster, "거래량"=→"거래량 27":waveform(dbl), "가격"=→"가격 27":waveform(i32), "참조 번호 출력"=w442:T2, "출력"=→"출력 27":T1)  [unwired: 4 in]
        n178 = Or(x=w440, y="정지 27") -> (x .or. y?=w438:bool)
        "run 27" <- w437
      }
      n179 = while {
        shift-right: [w418] -> w386
        shift-left: w388 -> [w419]
        shift-right: [w416] -> w385
        shift-left: w387 -> [w417]
        i -> [w413]
        stop <- w414 stop-if-true
        n180 = Wait (ms)(milliseconds to wait=u32 1000 ("대기 시간 (ms)")) -> ()  [unwired: 1 out]
        n181 = call "analysis_01(SubVI).vi"("에러 입력(에러 없음)"=w417, "품   번"="품   번 25", "참조 번호 입력"=w419) -> ("에러 출력"=w416:errorcluster, "거래량"=→"거래량 25":waveform(dbl), "가격"=→"가격 25":waveform(i32), "참조 번호 출력"=w418:T2, "출력"=→"출력 25":T1)  [unwired: 4 in]
        n182 = Or(x=w416, y="정지 25") -> (x .or. y?=w414:bool)
        "run 25" <- w413
      }
      n183 = call <vilib>:"CloseHandle.vi"("client handle"=w402, "error in (no error)"=w401) -> ()  [unwired: 13 in, 1 out]
      n184 = call <vilib>:"CloseHandle.vi"("client handle"=w399, "error in (no error)"=w400) -> ()  [unwired: 13 in, 1 out]
      n185 = call <vilib>:"CloseHandle.vi"("client handle"=w386, "error in (no error)"=w385) -> ()  [unwired: 13 in, 1 out]
    }
  }
  n186 = flat-sequence {
    frame #0 {
      n187 = local write item#16(FALSE ("clean")) -> ()
      n188 = local write item#30(FALSE ("clean")) -> ()
      n189 = local write item#6(FALSE ("clean")) -> ()
      n190 = case shown="참" "?" {
        frame False {
        }
        frame True {
          w495 = waveform(i32)[] [] ("히스토리 데이터")
          n191 = property on="가격 4" class="WFChart (엄격한)"("History Data"=w495) -> ()  [unwired: 2 in, 2 out]
          n192 = property on="거래량 4" class="WFChart (엄격한)"("History Data"=w495) -> ()  [unwired: 2 in, 2 out]
        }
      }
      n193 = case shown="참" "?" {
        frame False {
        }
        frame True {
          w494 = waveform(i32)[] [] ("히스토리 데이터")
          n194 = property on="가격 6" class="WFChart (엄격한)"("History Data"=w494) -> ()  [unwired: 2 in, 2 out]
          n195 = property on="거래량 6" class="WFChart (엄격한)"("History Data"=w494) -> ()  [unwired: 2 in, 2 out]
        }
      }
      n196 = case shown="참" "?" {
        frame False {
        }
        frame True {
          w498 = waveform(i32)[] [] ("히스토리 데이터")
          n197 = property on="가격" class="WFChart (엄격한)"("History Data"=w498) -> ()  [unwired: 2 in, 2 out]
          n198 = property on="거래량" class="WFChart (엄격한)"("History Data"=w498) -> ()  [unwired: 2 in, 2 out]
        }
      }
      n199 = local write item#7(FALSE ("clean")) -> ()
      n200 = local write item#29(FALSE ("clean")) -> ()
      n201 = local write item#15(FALSE ("clean")) -> ()
      n202 = case shown="참" "?" {
        frame False {
        }
        frame True {
          w497 = waveform(i32)[] [] ("히스토리 데이터")
          n203 = property on="가격 2" class="WFChart (엄격한)"("History Data"=w497) -> ()  [unwired: 2 in, 2 out]
          n204 = property on="거래량 2" class="WFChart (엄격한)"("History Data"=w497) -> ()  [unwired: 2 in, 2 out]
        }
      }
      n205 = case shown="참" "?" {
        frame False {
        }
        frame True {
          w493 = waveform(i32)[] [] ("히스토리 데이터")
          n206 = property on="가격 5" class="WFChart (엄격한)"("History Data"=w493) -> ()  [unwired: 2 in, 2 out]
          n207 = property on="거래량 5" class="WFChart (엄격한)"("History Data"=w493) -> ()  [unwired: 2 in, 2 out]
        }
      }
      n208 = case shown="참" "?" {
        frame False {
        }
        frame True {
          w496 = waveform(i32)[] [] ("히스토리 데이터")
          n209 = property on="가격 3" class="WFChart (엄격한)"("History Data"=w496) -> ()  [unwired: 2 in, 2 out]
          n210 = property on="거래량 3" class="WFChart (엄격한)"("History Data"=w496) -> ()  [unwired: 2 in, 2 out]
        }
      }
    }
  }
  n211 = flat-sequence {
    frame #0 {
      n212 = local write item#81(FALSE ("clean")) -> ()
      n213 = local write item#80(FALSE ("clean")) -> ()
      n214 = local write item#84(FALSE ("clean")) -> ()
      n215 = case shown="참" "?" {
        frame False {
        }
        frame True {
          w513 = waveform(i32)[] [] ("히스토리 데이터")
          n216 = property on="가격 10" class="WFChart (엄격한)"("History Data"=w513) -> ()  [unwired: 2 in, 2 out]
          n217 = property on="거래량 10" class="WFChart (엄격한)"("History Data"=w513) -> ()  [unwired: 2 in, 2 out]
        }
      }
      n218 = case shown="참" "?" {
        frame False {
        }
        frame True {
          w512 = waveform(i32)[] [] ("히스토리 데이터")
          n219 = property on="가격 8" class="WFChart (엄격한)"("History Data"=w512) -> ()  [unwired: 2 in, 2 out]
          n220 = property on="거래량 8" class="WFChart (엄격한)"("History Data"=w512) -> ()  [unwired: 2 in, 2 out]
        }
      }
      n221 = case shown="참" "?" {
        frame False {
        }
        frame True {
          w516 = waveform(i32)[] [] ("히스토리 데이터")
          n222 = property on="가격 12" class="WFChart (엄격한)"("History Data"=w516) -> ()  [unwired: 2 in, 2 out]
          n223 = property on="거래량 12" class="WFChart (엄격한)"("History Data"=w516) -> ()  [unwired: 2 in, 2 out]
        }
      }
      n224 = local write item#83(FALSE ("clean")) -> ()
      n225 = local write item#79(FALSE ("clean")) -> ()
      n226 = local write item#82(FALSE ("clean")) -> ()
      n227 = case shown="참" "?" {
        frame False {
        }
        frame True {
          w515 = waveform(i32)[] [] ("히스토리 데이터")
          n228 = property on="가격 11" class="WFChart (엄격한)"("History Data"=w515) -> ()  [unwired: 2 in, 2 out]
          n229 = property on="거래량 11" class="WFChart (엄격한)"("History Data"=w515) -> ()  [unwired: 2 in, 2 out]
        }
      }
      n230 = case shown="참" "?" {
        frame False {
        }
        frame True {
          w511 = waveform(i32)[] [] ("히스토리 데이터")
          n231 = property on="가격 7" class="WFChart (엄격한)"("History Data"=w511) -> ()  [unwired: 2 in, 2 out]
          n232 = property on="거래량 7" class="WFChart (엄격한)"("History Data"=w511) -> ()  [unwired: 2 in, 2 out]
        }
      }
      n233 = case shown="참" "?" {
        frame False {
        }
        frame True {
          w514 = waveform(i32)[] [] ("히스토리 데이터")
          n234 = property on="가격 9" class="WFChart (엄격한)"("History Data"=w514) -> ()  [unwired: 2 in, 2 out]
          n235 = property on="거래량 9" class="WFChart (엄격한)"("History Data"=w514) -> ()  [unwired: 2 in, 2 out]
        }
      }
    }
  }
  n236 = flat-sequence {
    frame #0 {
      n237 = local write item#123(FALSE ("clean")) -> ()
      n238 = local write item#122(FALSE ("clean")) -> ()
      n239 = local write item#126(FALSE ("clean")) -> ()
      n240 = case shown="참" "?" {
        frame False {
        }
        frame True {
          w531 = waveform(i32)[] [] ("히스토리 데이터")
          n241 = property on="가격 16" class="WFChart (엄격한)"("History Data"=w531) -> ()  [unwired: 2 in, 2 out]
          n242 = property on="거래량 16" class="WFChart (엄격한)"("History Data"=w531) -> ()  [unwired: 2 in, 2 out]
        }
      }
      n243 = case shown="참" "?" {
        frame False {
        }
        frame True {
          w530 = waveform(i32)[] [] ("히스토리 데이터")
          n244 = property on="가격 14" class="WFChart (엄격한)"("History Data"=w530) -> ()  [unwired: 2 in, 2 out]
          n245 = property on="거래량 14" class="WFChart (엄격한)"("History Data"=w530) -> ()  [unwired: 2 in, 2 out]
        }
      }
      n246 = case shown="참" "?" {
        frame False {
        }
        frame True {
          w534 = waveform(i32)[] [] ("히스토리 데이터")
          n247 = property on="가격 18" class="WFChart (엄격한)"("History Data"=w534) -> ()  [unwired: 2 in, 2 out]
          n248 = property on="거래량 18" class="WFChart (엄격한)"("History Data"=w534) -> ()  [unwired: 2 in, 2 out]
        }
      }
      n249 = local write item#125(FALSE ("clean")) -> ()
      n250 = local write item#121(FALSE ("clean")) -> ()
      n251 = local write item#124(FALSE ("clean")) -> ()
      n252 = case shown="참" "?" {
        frame False {
        }
        frame True {
          w533 = waveform(i32)[] [] ("히스토리 데이터")
          n253 = property on="가격 17" class="WFChart (엄격한)"("History Data"=w533) -> ()  [unwired: 2 in, 2 out]
          n254 = property on="거래량 17" class="WFChart (엄격한)"("History Data"=w533) -> ()  [unwired: 2 in, 2 out]
        }
      }
      n255 = case shown="참" "?" {
        frame False {
        }
        frame True {
          w529 = waveform(i32)[] [] ("히스토리 데이터")
          n256 = property on="가격 13" class="WFChart (엄격한)"("History Data"=w529) -> ()  [unwired: 2 in, 2 out]
          n257 = property on="거래량 13" class="WFChart (엄격한)"("History Data"=w529) -> ()  [unwired: 2 in, 2 out]
        }
      }
      n258 = case shown="참" "?" {
        frame False {
        }
        frame True {
          w532 = waveform(i32)[] [] ("히스토리 데이터")
          n259 = property on="가격 15" class="WFChart (엄격한)"("History Data"=w532) -> ()  [unwired: 2 in, 2 out]
          n260 = property on="거래량 15" class="WFChart (엄격한)"("History Data"=w532) -> ()  [unwired: 2 in, 2 out]
        }
      }
    }
  }
  n261 = flat-sequence {
    frame #0 {
      n262 = local write item#165(FALSE ("clean")) -> ()
      n263 = local write item#164(FALSE ("clean")) -> ()
      n264 = local write item#168(FALSE ("clean")) -> ()
      n265 = case shown="참" "?" {
        frame False {
        }
        frame True {
          w549 = waveform(i32)[] [] ("히스토리 데이터")
          n266 = property on="가격 22" class="WFChart (엄격한)"("History Data"=w549) -> ()  [unwired: 2 in, 2 out]
          n267 = property on="거래량 22" class="WFChart (엄격한)"("History Data"=w549) -> ()  [unwired: 2 in, 2 out]
        }
      }
      n268 = case shown="참" "?" {
        frame False {
        }
        frame True {
          w548 = waveform(i32)[] [] ("히스토리 데이터")
          n269 = property on="가격 20" class="WFChart (엄격한)"("History Data"=w548) -> ()  [unwired: 2 in, 2 out]
          n270 = property on="거래량 20" class="WFChart (엄격한)"("History Data"=w548) -> ()  [unwired: 2 in, 2 out]
        }
      }
      n271 = case shown="참" "?" {
        frame False {
        }
        frame True {
          w552 = waveform(i32)[] [] ("히스토리 데이터")
          n272 = property on="가격 24" class="WFChart (엄격한)"("History Data"=w552) -> ()  [unwired: 2 in, 2 out]
          n273 = property on="거래량 24" class="WFChart (엄격한)"("History Data"=w552) -> ()  [unwired: 2 in, 2 out]
        }
      }
      n274 = local write item#167(FALSE ("clean")) -> ()
      n275 = local write item#163(FALSE ("clean")) -> ()
      n276 = local write item#166(FALSE ("clean")) -> ()
      n277 = case shown="참" "?" {
        frame False {
        }
        frame True {
          w551 = waveform(i32)[] [] ("히스토리 데이터")
          n278 = property on="가격 23" class="WFChart (엄격한)"("History Data"=w551) -> ()  [unwired: 2 in, 2 out]
          n279 = property on="거래량 23" class="WFChart (엄격한)"("History Data"=w551) -> ()  [unwired: 2 in, 2 out]
        }
      }
      n280 = case shown="참" "?" {
        frame False {
        }
        frame True {
          w547 = waveform(i32)[] [] ("히스토리 데이터")
          n281 = property on="가격 19" class="WFChart (엄격한)"("History Data"=w547) -> ()  [unwired: 2 in, 2 out]
          n282 = property on="거래량 19" class="WFChart (엄격한)"("History Data"=w547) -> ()  [unwired: 2 in, 2 out]
        }
      }
      n283 = case shown="참" "?" {
        frame False {
        }
        frame True {
          w550 = waveform(i32)[] [] ("히스토리 데이터")
          n284 = property on="가격 21" class="WFChart (엄격한)"("History Data"=w550) -> ()  [unwired: 2 in, 2 out]
          n285 = property on="거래량 21" class="WFChart (엄격한)"("History Data"=w550) -> ()  [unwired: 2 in, 2 out]
        }
      }
    }
  }
  n286 = flat-sequence {
    frame #0 {
      n287 = local write item#207(FALSE ("clean")) -> ()
      n288 = local write item#206(FALSE ("clean")) -> ()
      n289 = local write item#210(FALSE ("clean")) -> ()
      n290 = case shown="참" "?" {
        frame False {
        }
        frame True {
          w567 = waveform(i32)[] [] ("히스토리 데이터")
          n291 = property on="가격 28" class="WFChart (엄격한)"("History Data"=w567) -> ()  [unwired: 2 in, 2 out]
          n292 = property on="거래량 28" class="WFChart (엄격한)"("History Data"=w567) -> ()  [unwired: 2 in, 2 out]
        }
      }
      n293 = case shown="참" "?" {
        frame False {
        }
        frame True {
          w566 = waveform(i32)[] [] ("히스토리 데이터")
          n294 = property on="가격 26" class="WFChart (엄격한)"("History Data"=w566) -> ()  [unwired: 2 in, 2 out]
          n295 = property on="거래량 26" class="WFChart (엄격한)"("History Data"=w566) -> ()  [unwired: 2 in, 2 out]
        }
      }
      n296 = case shown="참" "?" {
        frame False {
        }
        frame True {
          w570 = waveform(i32)[] [] ("히스토리 데이터")
          n297 = property on="가격 30" class="WFChart (엄격한)"("History Data"=w570) -> ()  [unwired: 2 in, 2 out]
          n298 = property on="거래량 30" class="WFChart (엄격한)"("History Data"=w570) -> ()  [unwired: 2 in, 2 out]
        }
      }
      n299 = local write item#209(FALSE ("clean")) -> ()
      n300 = local write item#205(FALSE ("clean")) -> ()
      n301 = local write item#208(FALSE ("clean")) -> ()
      n302 = case shown="참" "?" {
        frame False {
        }
        frame True {
          w569 = waveform(i32)[] [] ("히스토리 데이터")
          n303 = property on="가격 29" class="WFChart (엄격한)"("History Data"=w569) -> ()  [unwired: 2 in, 2 out]
          n304 = property on="거래량 29" class="WFChart (엄격한)"("History Data"=w569) -> ()  [unwired: 2 in, 2 out]
        }
      }
      n305 = case shown="참" "?" {
        frame False {
        }
        frame True {
          w565 = waveform(i32)[] [] ("히스토리 데이터")
          n306 = property on="가격 25" class="WFChart (엄격한)"("History Data"=w565) -> ()  [unwired: 2 in, 2 out]
          n307 = property on="거래량 25" class="WFChart (엄격한)"("History Data"=w565) -> ()  [unwired: 2 in, 2 out]
        }
      }
      n308 = case shown="참" "?" {
        frame False {
        }
        frame True {
          w568 = waveform(i32)[] [] ("히스토리 데이터")
          n309 = property on="가격 27" class="WFChart (엄격한)"("History Data"=w568) -> ()  [unwired: 2 in, 2 out]
          n310 = property on="거래량 27" class="WFChart (엄격한)"("History Data"=w568) -> ()  [unwired: 2 in, 2 out]
        }
      }
    }
  }
